vi "PID_controller.vi"(6 "PID gains":T1={"proportional gain (Kc)"=1.0, "integral time (Ti, min)"=0.01, "derivative time (Td, min)"=0.0} {"derivative time (Td, min)" format="%.3f"; "integral time (Ti, min)" format="%.3f"; "proportional gain (Kc)" format="%.3f"}, 9 "Setpoint":dbl format="%.2f", 11 "Process Variable":dbl format="%.2f") -> (1 "Direction":bool, 3 "output":dbl, 4 "dt out (s)":dbl format="%.3f", 5 "PreScaled O/P":dbl format="%.2f")   [LabVIEW 2021]
uses:
  <vilib>/addons/control/pid/pid.llb/PID (DBL).vi
  <vilib>/addons/control/pid/NI_PID_pid.lvlib
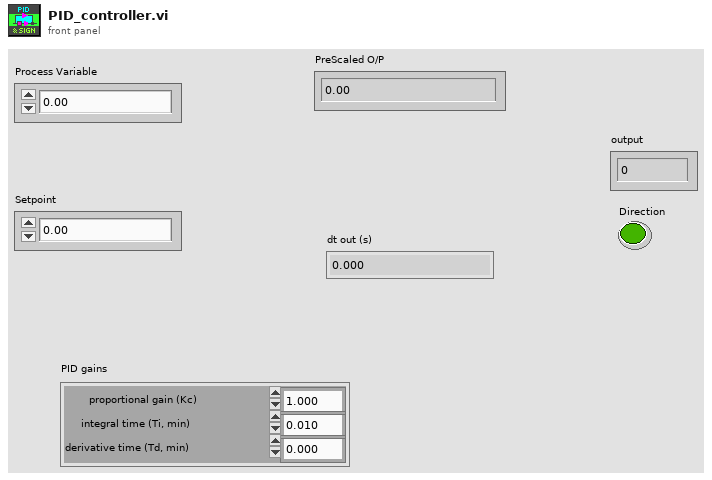
[diagram p1: front panel]
types:
  T1 = cluster{"proportional gain (Kc)":dbl, "integral time (Ti, min)":dbl, "derivative time (Td, min)":dbl}
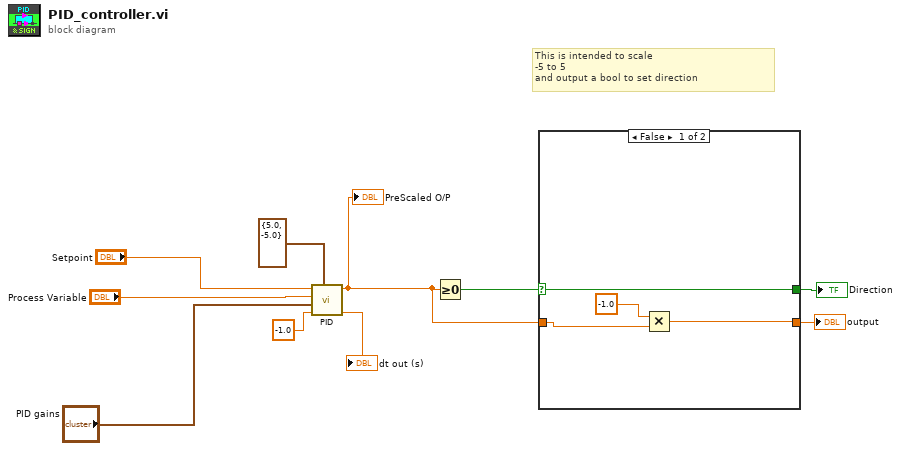
[diagram p0: block diagram]
diagram:
  # "This is intended to scale\n-5 to 5\nand output a bool to set direction"
  n1 = call-poly <vilib>:"PID.vi"("output range"=cluster{"output high":dbl, "output low":dbl} {"output high"=5.0, "output low"=-5.0}, "dt (s)"=-1.0, "PID gains"="PID gains", "process variable"="Process Variable", "setpoint"="Setpoint") -> ("dt out (s)"=→"dt out (s)":dbl, "output"=w4:dbl)  [unwired: 5 in]
  "PreScaled O/P" <- w4
  n2 = Greater Or Equal To 0?(x=w4) -> (x >= 0?=w5:bool)
  n3 = case shown="False" w5 {
    selector: w5 -> [w11 w15]
    tunnel: [w12 w16] -> w3
    tunnel: w4 -> [w14 w16]
    tunnel: [w11 w15] -> w2
    frame False {
      n4 = Multiply(x=-1.0, y=w14) -> (x*y=w12:dbl)
    }
    frame True {
    }
  }
  "output" <- w3
  "Direction" <- w2
